vi "moban.vi"   [LabVIEW 2017]
uses:
  <vilib>/MediaMongrels Ltd/WebSockets/WebSockets/WebSocket Client/WebSocket Client.lvclass
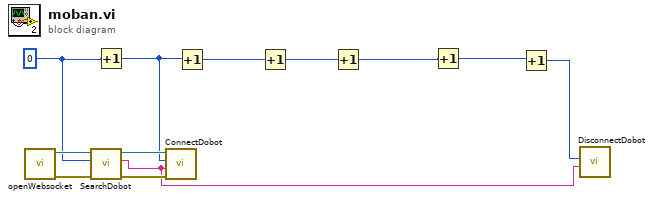
[diagram p0: block diagram]
diagram:
  w8 = 0 ("id")
  n1 = call <vilib>:"openWebsocket.vi"() -> ("error out"=w10:errorcluster, "WebSocket Client out"=w12:refnum<class "WebSocket Client.lvclass">)  [unwired: 10 in]
  n2 = call <vilib>:"SearchDobot.vi"("error in (no error)"=w10, "id"=w8, "WebSocket in"=w12) -> ("error out"=w9:errorcluster, "portName"=w1:string, "WebSocket out"=w11:refnum<class "WebSocket Client.lvclass">)  [unwired: 6 in]
  n3 = Increment(x=w8) -> (x+1=w7:i32)
  n4 = call <vilib>:"ConnectDobot.vi"("error in (no error)"=w9, "portName"=w1, "id"=w7, "WebSocket in"=w11) -> ()  [unwired: 5 in, 3 out]
  n5 = Increment(x=w7) -> (x+1=w5:i32)
  n6 = Increment(x=w5) -> (x+1=w4:i32)
  n7 = Increment(x=w4) -> (x+1=w3:i32)
  n8 = Increment(x=w3) -> (x+1=w2:i32)
  n9 = Increment(x=w2) -> (x+1=w6:i32)
  n10 = call <vilib>:"DisconnectDobot.vi"("portName"=w1, "id"=w6) -> ()  [unwired: 7 in, 3 out]
